vi "Read Integral accumulator.vi"(8 "error in (no error)":errorcluster, 11 "PID Control in":refnum<class "PID Control.lvclass">) -> (0 "error out":errorcluster, 2 "Integral accumulator":dbl, 3 "PID Control out":refnum<class "PID Control.lvclass">)   [LabVIEW 2016, in "PID Control.lvclass"]
uses:
  PID Control.lvclass
  PID Control.lvclass/PID Control.ctl
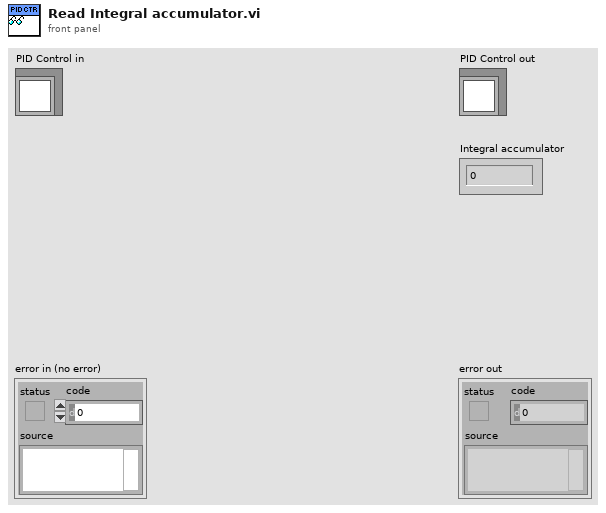
[diagram p1: front panel]
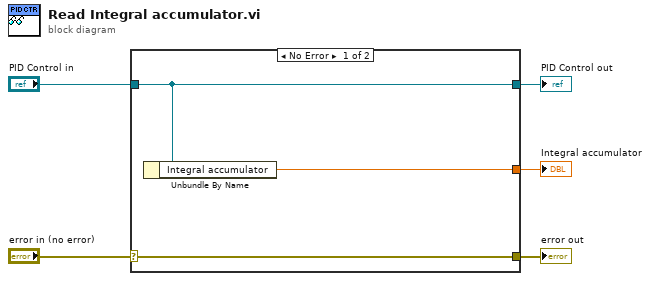
[diagram p0: block diagram]
diagram:
  n1 = case shown="No Error" "error in (no error)" {
    selector: "error in (no error)" -> [w8 w9]
    tunnel: [w8 w9] -> w4
    tunnel: [w7 w10] -> w2
    tunnel: "PID Control in" -> [w7 w10]
    tunnel: [w6 _] -> w1
    frame No Error {
      n2 = Unbundle By Name(w7) -> ("Integral accumulator"=w6:dbl)
    }
    frame Error {
    }
  }
  "error out" <- w4
  "PID Control out" <- w2
  "Integral accumulator" <- w1
